vi "Controller Apply Soft Configuration.vi"(8 "error in (no error)":errorcluster, 11 "FOFB Configuration":T1={"FOFB Parameters"={"Network"={"FOFB Controller IP"="", "LNLS Control Network IP"="", "LNLS Control Network Power Supplies TCP Port"=0, "LNLS Control Network FOFB Configuration TCP Port"=0, "LNLS Control Network BPMs TCP Port"=0, "Data Server TCP Port"=0, "Monitoring Data TCP Port"=0, "Configuration GUI TCP Port"=0, "Storage Data TCP Port"=0, "Fast Command TCP Port"=0, "TCP Listening Timeout"=0, "Request Setpoints Rate"=0}, "Fast Acquisition"={"Acquisition Period"=0, "Data Buffer Size"=0, "Monitoring Period"=0}, "Response Matrix Measurement"={"Step Amplitude"=0.0, "Time Between Steps"=0, "Step Duration"=0, "Number of Averages"=0}, "Correction Algorithm"={"Correction Period"=0, "Reference Orbit Path"=path "", "Response Matrix Path"=path "", "Correction Matrix Path"=path "", "PID Horizontal Gain"=0.0, "PID Vertical Gain"=0.0, "PID Horizontal Integral Time"=0.0, "PID Vertical Integral Time"=0.0, "PID Horizontal Derivative Time"=0.0, "PID Vertical Derivative Time"=0.0, "Beam Current FOFB Threshold"=0.0, "Decouple H-V"=FALSE, "Use Additional BPM LPF"=FALSE, "BPM LPF Cutoff"=0.0}, "Acquisition Network"=[], "Actuation Network"=[]}, "Number of Acquisition Chassis"=0, "Number of Actuation Chassis"=0, "Number of BPM Readings"=0, "BPM Reading Names"=[], "Selected BPM Readings"=[0, 1, 2, 3, 4, 5, 6, 7, 8, 9, 10, 11, 12, 13, 14, 15, 16, 17, 18, 19, 20, 21, 22, 23, 24, 25, 26, 27, 28, 29, 30, 31, 32, 33, 34, 35, 36, 37, 38, 39, 40, 41, 42, 43, 44, 45, 46, 47, 48, 49], "Number of Correctors"=0, "Corrector Names"=[], "Selected Correctors"=[0, 1, 2, 3, 4, 5, 6, 7, 8, 9, 10, 11, 12, 13, 14, 15, 16, 17, 18, 19, 20, 21, 22, 23, 24, 25, 26, 27, 28, 29, 30, 31, 32, 33, 34, 35, 36, 37, 38, 39, 40, 41, 42, 43, 44, 45, 46, 47, 48, 49], "Reference Orbit"=[], "Response Matrix"=[], "Correction Matrix"=[], "Acquisition Chassis Names"=[], "Actuation Chassis Names"=[], "Acquisition Variables"=[], "Actuation Variables"=[], "PS Matrix Mapping"=[], "Inverse PS Matrix Mapping"=[], "BPM Matrix Mapping"=[], "Inverse BPM Matrix Mapping"=[], "Response Matrix Beam Energy (MeV)"=0.0, "PID Parameters"=[], "BPM Planes"=[], "Corrector Planes"=[], "RMM Step Factor"=[]}) -> (0 "error out":errorcluster, 3 "FOFB Configuration":T1={"FOFB Parameters"={"Network"={"FOFB Controller IP"="", "LNLS Control Network IP"="", "LNLS Control Network Power Supplies TCP Port"=0, "LNLS Control Network FOFB Configuration TCP Port"=0, "LNLS Control Network BPMs TCP Port"=0, "Data Server TCP Port"=0, "Monitoring Data TCP Port"=0, "Configuration GUI TCP Port"=0, "Storage Data TCP Port"=0, "Fast Command TCP Port"=0, "TCP Listening Timeout"=0, "Request Setpoints Rate"=0}, "Fast Acquisition"={"Acquisition Period"=0, "Data Buffer Size"=0, "Monitoring Period"=0}, "Response Matrix Measurement"={"Step Amplitude"=0.0, "Time Between Steps"=0, "Step Duration"=0, "Number of Averages"=0}, "Correction Algorithm"={"Correction Period"=0, "Reference Orbit Path"=path "", "Response Matrix Path"=path "", "Correction Matrix Path"=path "", "PID Horizontal Gain"=0.0, "PID Vertical Gain"=0.0, "PID Horizontal Integral Time"=0.0, "PID Vertical Integral Time"=0.0, "PID Horizontal Derivative Time"=0.0, "PID Vertical Derivative Time"=0.0, "Beam Current FOFB Threshold"=0.0, "Decouple H-V"=FALSE, "Use Additional BPM LPF"=FALSE, "BPM LPF Cutoff"=0.0}, "Acquisition Network"=[], "Actuation Network"=[]}, "Number of Acquisition Chassis"=0, "Number of Actuation Chassis"=0, "Number of BPM Readings"=0, "BPM Reading Names"=[], "Selected BPM Readings"=[0, 1, 2, 3, 4, 5, 6, 7, 8, 9, 10, 11, 12, 13, 14, 15, 16, 17, 18, 19, 20, 21, 22, 23, 24, 25, 26, 27, 28, 29, 30, 31, 32, 33, 34, 35, 36, 37, 38, 39, 40, 41, 42, 43, 44, 45, 46, 47, 48, 49], "Number of Correctors"=0, "Corrector Names"=[], "Selected Correctors"=[0, 1, 2, 3, 4, 5, 6, 7, 8, 9, 10, 11, 12, 13, 14, 15, 16, 17, 18, 19, 20, 21, 22, 23, 24, 25, 26, 27, 28, 29, 30, 31, 32, 33, 34, 35, 36, 37, 38, 39, 40, 41, 42, 43, 44, 45, 46, 47, 48, 49], "Reference Orbit"=[], "Response Matrix"=[], "Correction Matrix"=[], "Acquisition Chassis Names"=[], "Actuation Chassis Names"=[], "Acquisition Variables"=[], "Actuation Variables"=[], "PS Matrix Mapping"=[], "Inverse PS Matrix Mapping"=[], "BPM Matrix Mapping"=[], "Inverse BPM Matrix Mapping"=[], "Response Matrix Beam Energy (MeV)"=0.0, "PID Parameters"=[], "BPM Planes"=[], "Corrector Planes"=[], "RMM Step Factor"=[]})   [LabVIEW 2011, in "Controller VIs.lvlib"]
doc: "Performs tasks related with the FOFB configuration which does not require interrupting controller execution (ex.: load response matrix and reference orbit from file, calculate correction matrix, etc)."
uses:
  Controller VIs.lvlib
  Types Definitions/Type FOFB Configuration.ctl
  Types Definitions/Type FOFB Parameters.ctl
  Types Definitions/Type Network Configuration.ctl
  Types Definitions/Type FA Configuration.ctl
  Types Definitions/Type Response Matrix Measurement Configuration.ctl
  Types Definitions/Type Correction Algorithm Configuration.ctl
  Types Definitions/Type Acquisition Network Configuration.ctl
  Types Definitions/Type Actuation Network Configuration.ctl
  Types Definitions/Type PID Parameters.ctl
  File VIs.lvlib
  XML VIs.lvlib
  Simulated Beam VIs/Simulated Beam Response.vi
  Simulated Beam VIs.lvlib
  Simulated Beam VIs/Simulated PS Current.vi
  Type Definitions.lvlib
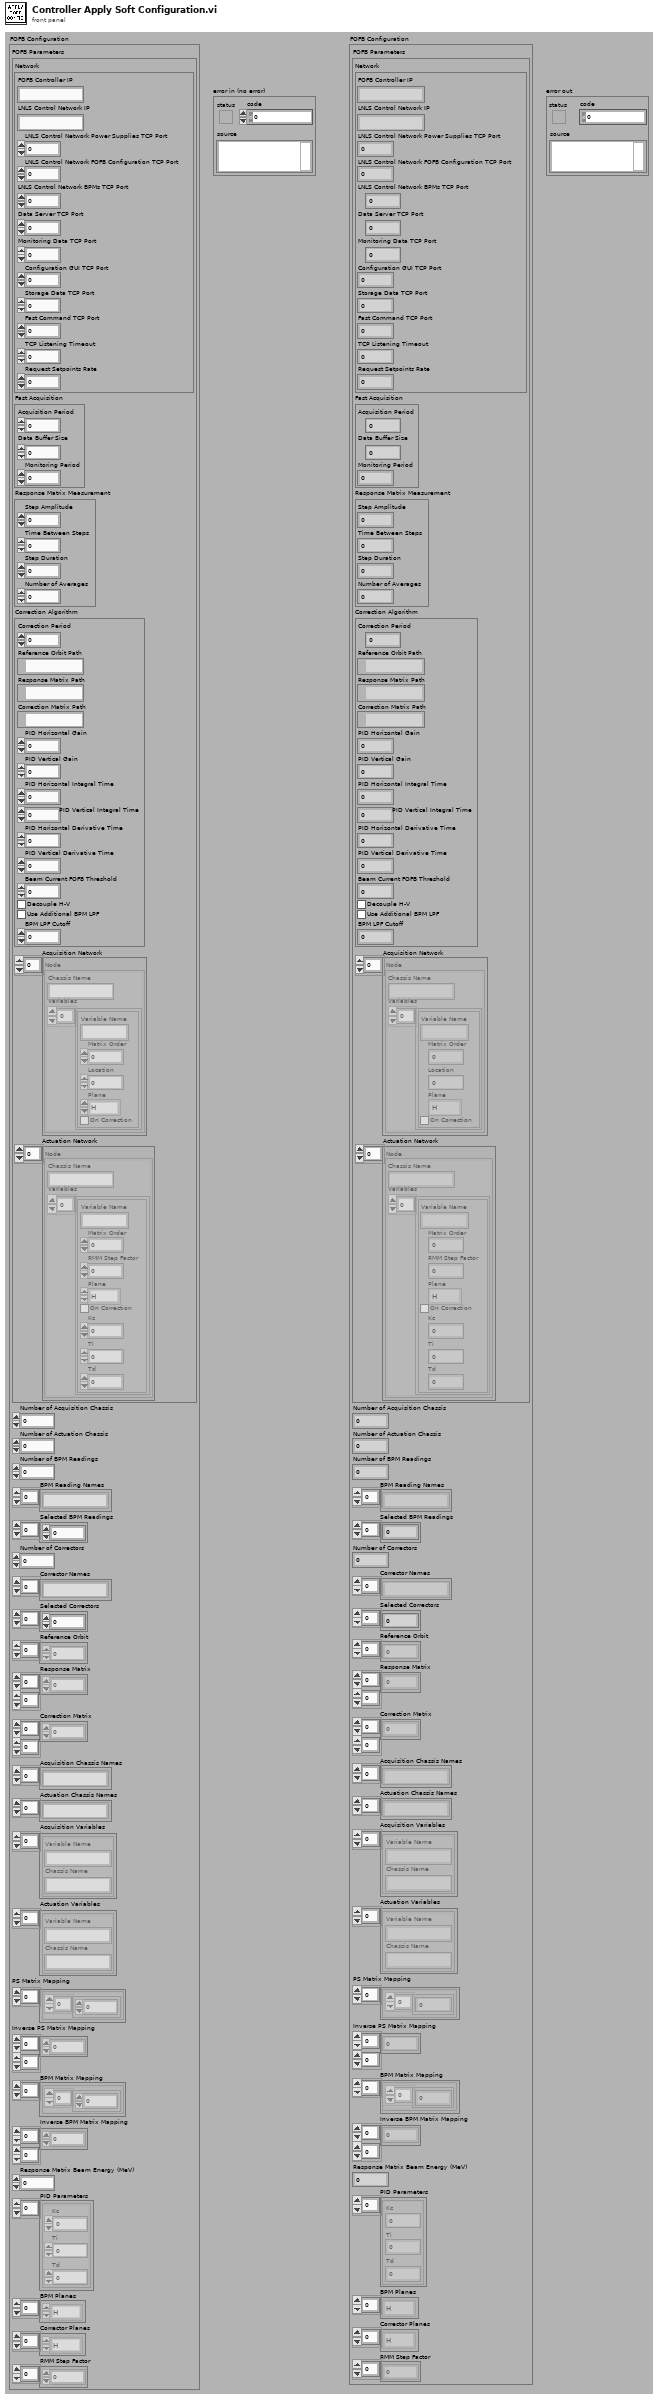
[diagram p1: front panel]
types:
  T1 = typedef "Type Definitions.lvlib/Type FOFB Configuration.ctl" = cluster{"FOFB Parameters":T2, "Number of Acquisition Chassis":i32, "Number of Actuation Chassis":i32, "Number of BPM Readings":i32, "BPM Reading Names":string[], "Selected BPM Readings":u32[], "Number of Correctors":i32, "Corrector Names":string[], "Selected Correctors":u32[], "Reference Orbit":dbl[], "Response Matrix":dbl[][], "Correction Matrix":dbl[][], "Acquisition Chassis Names":string[], "Actuation Chassis Names":string[], "Acquisition Variables":cluster{"Variable Name":string, "Chassis Name":string}[], "Actuation Variables":cluster{"Variable Name":string, "Chassis Name":string}[], "PS Matrix Mapping":cluster{u32[]}[], "Inverse PS Matrix Mapping":u32[][], "BPM Matrix Mapping":cluster{u32[]}[], "Inverse BPM Matrix Mapping":u32[][], "Response Matrix Beam Energy (MeV)":dbl, "PID Parameters":T9[], "BPM Planes":enum8{"H", "V"}[], "Corrector Planes":enum8{"H", "V"}[], "RMM Step Factor":dbl[]}
  T2 = typedef "Type Definitions.lvlib/Type FOFB Parameters.ctl" = cluster{"Network":T3, "Fast Acquisition":T4, "Response Matrix Measurement":T5, "Correction Algorithm":T6, "Acquisition Network":T7, "Actuation Network":T8}
  T3 = typedef "Type Definitions.lvlib/Type Network Configuration.ctl" = cluster{"FOFB Controller IP":string, "LNLS Control Network IP":string, "LNLS Control Network Power Supplies TCP Port":u16, "LNLS Control Network FOFB Configuration TCP Port":u16, "LNLS Control Network BPMs TCP Port":u16, "Data Server TCP Port":u16, "Monitoring Data TCP Port":u16, "Configuration GUI TCP Port":u16, "Storage Data TCP Port":u16, "Fast Command TCP Port":u16, "TCP Listening Timeout":i32, "Request Setpoints Rate":u16}
  T4 = typedef "Type Definitions.lvlib/Type FA Configuration.ctl" = cluster{"Acquisition Period":u32, "Data Buffer Size":u32, "Monitoring Period":u32}
  T5 = typedef "Type Definitions.lvlib/Type Response Matrix Measurement Configuration.ctl" = cluster{"Step Amplitude":dbl, "Time Between Steps":u32, "Step Duration":u32, "Number of Averages":u32}
  T6 = typedef "Type Definitions.lvlib/Type Correction Algorithm Configuration.ctl" = cluster{"Correction Period":u32, "Reference Orbit Path":path, "Response Matrix Path":path, "Correction Matrix Path":path, "PID Horizontal Gain":dbl, "PID Vertical Gain":dbl, "PID Horizontal Integral Time":dbl, "PID Vertical Integral Time":dbl, "PID Horizontal Derivative Time":dbl, "PID Vertical Derivative Time":dbl, "Beam Current FOFB Threshold":dbl, "Decouple H-V":bool, "Use Additional BPM LPF":bool, "BPM LPF Cutoff":dbl}
  T7 = typedef "Type Definitions.lvlib/Type Acquisition Network Configuration.ctl" = cluster{"Chassis Name":string, "Variables":cluster{"Variable Name":string, "Matrix Order":u32, "Location":dbl, "Plane":enum8{"H", "V"}, "On Correction":bool}[]}[]
  T8 = typedef "Type Definitions.lvlib/Type Actuation Network Configuration.ctl" = cluster{"Chassis Name":string, "Variables":cluster{"Variable Name":string, "Matrix Order":u32, "RMM Step Factor":dbl, "Plane":enum8{"H", "V"}, "On Correction":bool, "Kc":dbl, "Ti":dbl, "Td":dbl}[]}[]
  T9 = typedef "Type Definitions.lvlib/Type PID Parameters.ctl" = cluster{"Kc":fxp<+/-,16,8>, "Ti":fxp<+/-,16,8>, "Td":fxp<+/-,16,8>}
  T10 = typedef "Type Definitions.lvlib/Type BPM Parameters.ctl" = cluster{"Location":dbl, "Plane":enum8{"H", "V"}, "On Correction":bool}
  T11 = typedef "Type Definitions.lvlib/Type PS Parameters.ctl" = cluster{"RMM Step Factor":dbl, "Plane":enum8{"H", "V"}, "On Correction":bool}
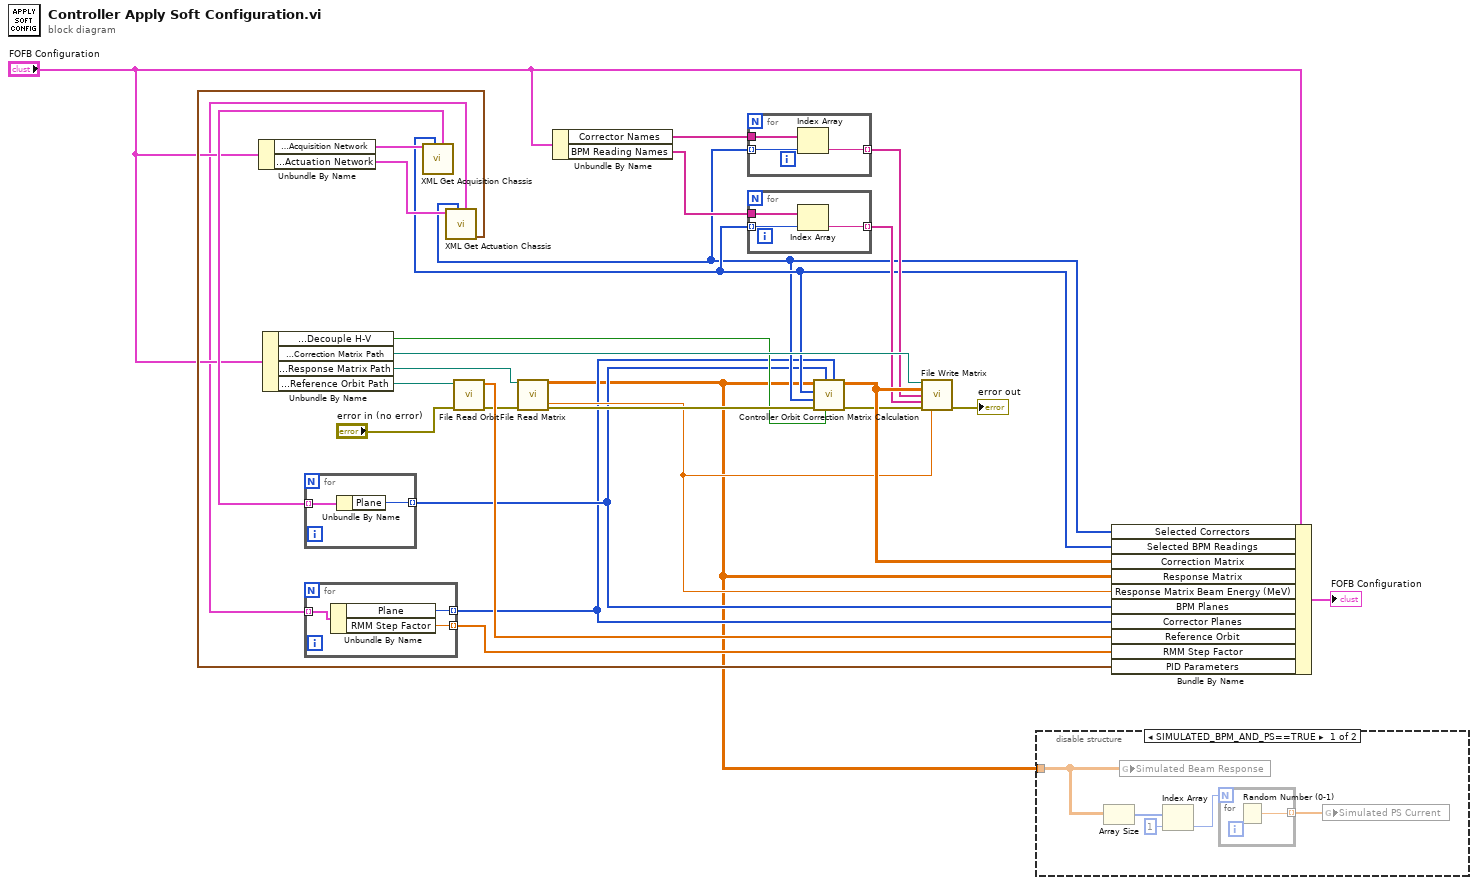
[diagram p0: block diagram]
diagram:
  n1 = Unbundle By Name("FOFB Configuration") -> ("FOFB Parameters.Acquisition Network"=w26:T7, "FOFB Parameters.Actuation Network"=w27:T8)
  n2 = Unbundle By Name("FOFB Configuration") -> ("FOFB Parameters.Correction Algorithm.Decouple H-V"=w7:bool, "FOFB Parameters.Correction Algorithm.Correction Matrix Path"=w15:path, "FOFB Parameters.Correction Algorithm.Response Matrix Path"=w20:path, "FOFB Parameters.Correction Algorithm.Reference Orbit Path"=w19:path)
  n3 = call "XML Get Acquisition Chassis.vi"("Acquisition Network"=w26) -> ("BPM Parameters"=w28:T10[], "Selected BPM Readings"=w6:u32[])  [unwired: 4 in, 5 out]
  n4 = for {
    tunnel: w28 -> [w31] mode=indexing
    tunnel: [w30] -> w3 mode=indexing
    n5 = Unbundle By Name(w31) -> ("Plane"=w30:enum8{"H", "V"})
  }
  n6 = call "XML Get Actuation Chassis.vi"("Actuation Network"=w27) -> ("PID Parameters"=w29:T9[], "PS Parameters"=w11:T11[], "Selected Correctors"=w5:u32[])  [unwired: 3 in, 5 out]
  n7 = for {
    tunnel: w11 -> [w34] mode=indexing
    tunnel: [w33] -> w2 mode=indexing
    tunnel: [w32] -> w4 mode=indexing
    n8 = Unbundle By Name(w34) -> ("Plane"=w33:enum8{"H", "V"}, "RMM Step Factor"=w32:dbl)
  }
  n9 = call "File Read Orbit.vi"("error in (no error)"="error in (no error)", "file path (dialog if empty)"=w19) -> ("error out"=w16:errorcluster, "Orbit"=w24:dbl[])  [unwired: 7 in, 1 out]
  n10 = call "File Read Matrix.vi"("file path (dialog if empty)"=w20, "error in (no error)"=w16) -> ("Matrix"=w1:dbl[][], "Beam Energy (MeV)"=w8:dbl, "error out"=w18:errorcluster)  [unwired: 9 in, 2 out]
  n11 = Unbundle By Name("FOFB Configuration") -> ("Corrector Names"=w12:string[], "BPM Reading Names"=w13:string[])
  n12 = for {
    tunnel: w5 -> [w36] mode=indexing
    tunnel: w12 -> [w37]
    tunnel: [w35] -> w9 mode=indexing
    n13 = Index Array(array=w37, index=w36) -> (element=w35:string)
  }
  n14 = for {
    tunnel: w6 -> [w39] mode=indexing
    tunnel: w13 -> [w40]
    tunnel: [w38] -> w10 mode=indexing
    n15 = Index Array(array=w40, index=w39) -> (element=w38:string)
  }
  n16 = call "Controller Orbit Correction Matrix Calculation.vi"("Corrector Planes"=w2, "Decouple H-V? (true)"=w7, "BPM Reading Planes"=w3, "error in (no error)"=w18, "Selected Correctors"=w5, "Selected BPM Readings"=w6, "Response Matrix"=w1) -> ("error out"=w17:errorcluster, "Correction Matrix"=w25:dbl[][])  [unwired: 3 in]
  n17 = call "File Write Matrix.vi"("file path (dialog if empty)"=w15, "Matrix"=w25, "Row Names"=w9, "Column Names"=w10, "error in (no error)"=w17, "Beam Energy (MeV)"=w8) -> ("error out"=→"error out":errorcluster)  [unwired: 9 in]
  n18 = disable-structure shown="SIMULATED_BPM_AND_PS==TRUE" {
    disable-tunnel: w1 -> [w45 _]
    frame condition #0 {
      n19 = Array Size(array=w45) -> (size(s)=w44:i32[])
      n20 = global write "Simulated Beam Response.vi" "Simulated Beam Response"(w45) -> ()
      n21 = Index Array(array=w44, index=1) -> (element=w42:i32)
      n22 = for {
        N: w42 -> [_]
        tunnel: [w46] -> w41 mode=indexing
        n23 = Random Number (0-1)() -> (number: 0 to 1=w46:dbl)
      }
      n24 = global write "Simulated PS Current.vi" "Simulated PS Current"(w41) -> ()
    }
    frame condition #1 (active) {
    }
  }
  n25 = Bundle By Name(cluster="FOFB Configuration", "Selected Correctors"=w5, "Selected BPM Readings"=w6, "Correction Matrix"=w25, "Response Matrix"=w1, "Response Matrix Beam Energy (MeV)"=w8, "BPM Planes"=w3, "Corrector Planes"=w2, "Reference Orbit"=w24, "RMM Step Factor"=w4, "PID Parameters"=w29) -> (→"FOFB Configuration":T1)
